vi "Set Software Limit Configuration.vi"(4 "error in (no error)":errorcluster, 5 "Software limit Configuration":T1, 6 "Axis (1)":i32=1 min=1 max=3, 7 "VISA resource name":refnum<visa-resource-name>) -> (0 "error out":errorcluster, 3 "VISA resource name out":refnum<visa-resource-name>)   [LabVIEW 2019, in "Newport ESP301.lvlib"]
doc: "This command is used to set the software limit checking and event handling for axis specified with <B>Axis (1)</B>.\nNOTE: If bit-0 or both bits-1 and -2 are set to zero(0) then no action will be taken by the controller."
uses:
  Newport ESP301.lvlib
panel:
  # "reserved"
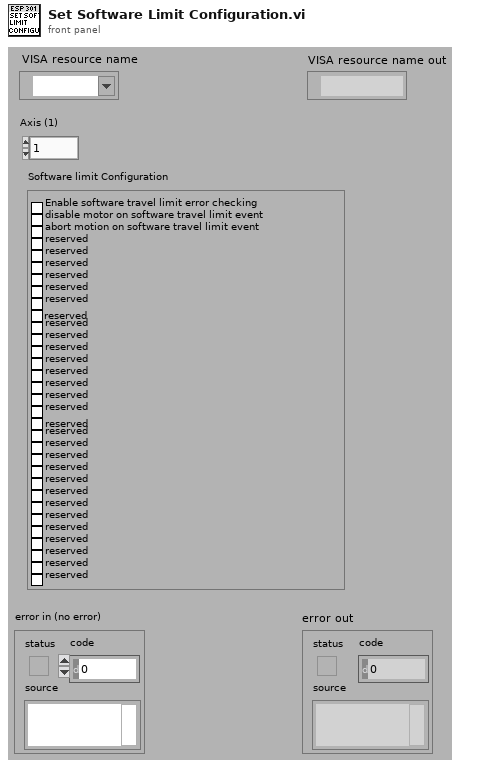
[diagram p1: front panel]
types:
  T1 = cluster{"Enable software travel limit error checking":bool, "disable motor on software travel limit event":bool, "abort motion on software travel limit event":bool, "reserved":bool, "reserved":bool, "reserved  ":bool, "reserved  ":bool, "reserved":bool, "reserved  ":bool, bool, "reserved":bool, "reserved":bool, "reserved ":bool, "reserved ":bool, "reserved":bool, "reserved ":bool, "reserved":bool, "reserved ":bool, "reserved ":bool, "reserved ":bool, "reserved ":bool, "reserved ":bool, "reserved ":bool, "reserved ":bool, "reserved ":bool, "reserved ":bool, "reserved ":bool, "reserved ":bool, "reserved ":bool, "reserved ":bool, "reserved ":bool, "reserved":bool}
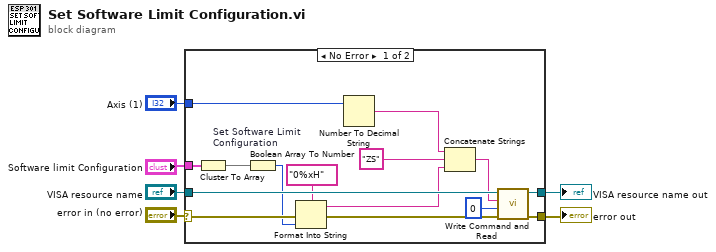
[diagram p0: block diagram]
diagram:
  n1 = case shown="No Error" "error in (no error)" {
    selector: "error in (no error)" -> [w12 w23]
    tunnel: [w20 w23] -> w6
    tunnel: "VISA resource name" -> [w21 w22]
    tunnel: [w19 w22] -> w5
    tunnel: "Axis (1)" -> [w15 _]
    tunnel: "Software limit Configuration" -> [w9 _]
    frame No Error {
      w18 = "ZS"  # Set Software Limit Configuration
      n2 = Cluster To Array(cluster=w9) -> (array=w13:bool[])
      n3 = Boolean Array To Number(Boolean array=w13) -> (number=w10:u32)
      n4 = Format Into String(format string="0%xH" ("chaîne de format"), error in=w12, w10) -> (resulting string=w8:string, error out=w11:errorcluster)  [unwired: 1 in]
      n5 = Number To Decimal String(number=w15) -> (decimal integer string=w14:string)  [unwired: 1 in]
      n6 = Concatenate Strings(w14, w18, w8) -> (w17:string)
      n7 = call "Write Command and Read.vi"("error in (no error)"=w11, "Bytes to read (100)"=u32 0, "Command"=w17, "VISA resource name"=w21) -> ("error out"=w20:errorcluster, "VISA resource name out"=w19:refnum<visa-resource-name>)  [unwired: 1 in, 3 out]
    }
    frame Error {
    }
  }
  "error out" <- w6
  "VISA resource name out" <- w5
